vi "robot_control.vi"() -> ()   [LabVIEW 2011]
uses:
  <vilib>/Rock Robotics/WPI/DriverStation/WPI_DriverStationRobotMode.ctl
  <vilib>/Rock Robotics/WPI/Solenoid/Deprecated/WPI_SolenoidSetBool.vi
  Robot Global Data.vi
  <vilib>/Rock Robotics/WPI/Solenoid/Deprecated/WPI_SolenoidGetBool.vi
  <vilib>/addons/control/pid/pid.llb/PID (DBL).vi
  <vilib>/Rock Robotics/WPI/RobotDrive/WPI_RobotDriveArcadeDrive_Standard(NoSaturation).vi
  <vilib>/addons/control/pid/NI_PID_pid.lvlib
  <vilib>/Rock Robotics/WPI/DriverStation/DriverStationLCD/WPI_DriverStationLCDLCDLine.ctl
panel:
  out "l rate":dbl
  out "l Distance":dbl
  out "r rate":dbl
  out "r Distance":dbl
  out "w index":bool
  out "s index":bool
  in  "reinitialize":bool
  out "i per ms":dbl
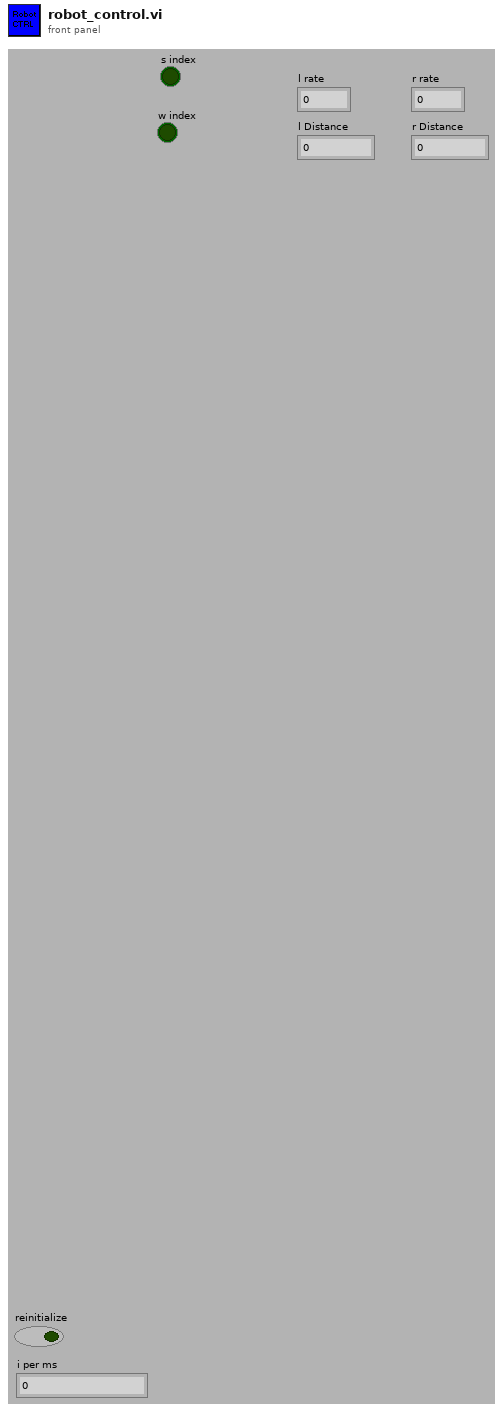
[diagram p1: front panel]
types:
  T1 = typedef "WPI_SolenoidDevRef.ctl" = cluster{"DevStatus":errorcluster, "Solenoid Module":T2, "Forward Solenoid Channel":T3, "Reverse Solenoid Channel":T3}
  T2 = typedef "FPGA_TypedefSolenoidModule.ctl" = enum16{"Solenoid Module 1", "Solenoid Module 2"}
  T3 = typedef "WPI_SolenoidChannel.ctl" = enum8{"Solenoid 1", "Solenoid 2", "Solenoid 3", "Solenoid 4", "Solenoid 5", "Solenoid 6", "Solenoid 7", "Solenoid 8", "Invalid"}
  T4 = typedef "WPI_DigitalInputDevRef.ctl" = cluster{"DevStatus":errorcluster, "DIO Channel":T5, "Digital Module":T6}
  T5 = typedef "FPGA_DIOChannel.ctl" = enum8{"DIO 1", "DIO 2", "DIO 3", "DIO 4", "DIO 5", "DIO 6", "DIO 7", "DIO 8", "DIO 9", "DIO 10", "DIO 11", "DIO 12", "DIO 13", "DIO 14", "Invalid"}
  T6 = typedef "FPGA_TypedefDigitalModule.ctl" = enum16{"Digital Module 1", "Digital Module 2"}
  T7 = typedef "WPI_EncoderDevRef.ctl" = cluster{"DevStatus":errorcluster, "EncoderIndex":T8, "CounterIndex":T9, "DistancePerCount":dbl, "Decoding Type":T10}
  T8 = typedef "FPGA_EncoderIdx.ctl" = enum8{"Enc 0", "Enc 1", "Enc 2", "Enc 3", "Invalid"}
  T9 = typedef "FPGA_CounterCtrSystemIndex.ctl" = enum8{"Ctr 0", "Ctr 1", "Ctr 2", "Ctr 3", "Ctr 4", "Ctr 5", "Ctr 6", "Ctr 7", "Invalid"}
  T10 = typedef "WPI_EncoderType.ctl" = enum16{"1x", "2x", "4x"}
  T11 = typedef "WPI_MotorControlDeviceRef.ctl" = cluster{"DeviceStatus":errorcluster, "Type":enum16{"PWM", "CAN"}, "PWM":cluster{"Digital Module":T6, "PWM Channel":T12, "DeadBand":T13}, "CAN":cluster{"Device Number":u8, "Control Mode":T14, "Semaphore":T15, "Max Vout":dbl}, "Invert":bool, "TransformRef":T16, "InvTransformRef":T16}
  T12 = typedef "FPGA_DIOPWMChannel.ctl" = enum8{"PWM 1", "PWM 2", "PWM 3", "PWM 4", "PWM 5", "PWM 6", "PWM 7", "PWM 8", "PWM 9", "PWM 10", "Invalid"}
  T13 = typedef "WPI_PWMDeadband.ctl" = cluster{"Name":string, "maxPositivePwm":i32, "minPositivePwm":i32, "centerPwm":i32, "maxNegativePwm":i32, "minNegativePwm":i32, "angularRange":u16}
  T14 = typedef "WPI_CANJaguar_ControlMode.ctl" = enum8{"Percent VBus", "Current", "Speed", "Position", "Voltage"}
  T15 = typedef "Semaphore RefNum" = refnum<k1>
  T16 = typedef "WPI_PWMTransform_ConPane.ctl" = refnum<vi>
  T17 = typedef "WPI_RobotDriveDevRef.ctl" = cluster{"DevStatus":errorcluster, "Motors[]":T11[], "Square Inputs":bool, "Max Output":dbl, "Isochronous":bool}
  T18 = typedef "WPI_DriverStationRobotMode.ctl" = enum16{"Autonomous Disabled", "Autonomous Enabled", "Teleop Disabled", "Teleop Enabled", "Timeout", "Finish"}
  T19 = typedef "WPI_DriverStationLCDLCDLine.ctl" = enum16{"Main - Line 1", "User - Line 2", "User - Line 3", "User - Line 4", "User - Line 5", "User - Line 6"}
  T20 = cluster{"proportional gain (Kc)":dbl, "integral time (Ti, min)":dbl, "derivative time (Td, min)":dbl}
  T21 = typedef "robot_control.ctl" = cluster{"Joystick1":cluster{"Buttons":T22, "Axes":cluster{"axis 1 (x)":dbl, "axis 2 (y)":dbl, "axis 3 (throttle)":dbl}}, "Joystick2":cluster{"Buttons":T22, "Axes":cluster{"axis 1 (x)":dbl, "axis 2 (y)":dbl, "axis 3 (throttle)":dbl}}, "Joystick3":cluster{"Buttons":T22, "Axes":cluster{"axis 1 (x)":dbl, "axis 2 (y)":dbl, "axis 3 (throttle)":dbl}}, "switchbox":cluster{"Driver Station Digital Input (1-8)[0]":bool, "Driver Station Digital Input (1-8)[1]":bool, "Driver Station Digital Input (1-8)[2]":bool, "Driver Station Digital Input (1-8)[3]":bool, "Driver Station Digital Input (1-8)[4]":bool, "Driver Station Digital Input (1-8)[5]":bool, "Driver Station Digital Input (1-8)[6]":bool, "Driver Station Digital Input (1-8)[7]":bool, "Driver Station Digital Input (1-8)[8]":bool}}
  T22 = typedef "WPI_JoystickButtonState.ctl" = cluster{"Button 1":bool, "Button 2":bool, "Button 3":bool, "Button 4":bool, "Button 5":bool, "Button 6":bool, "Button 7":bool, "Button 8":bool, "Button 9":bool, "Button 10":bool, "Button 11":bool, "Button 12":bool}
  T23 = typedef "match_data.ctl" = cluster{"Match Info":T24, "Derived Robot State":T25, "RobotMode":T18}
  T24 = typedef "WPI_DriverStationMatch Info.ctl" = cluster{"Autonomous Elapsed Seconds":dbl, "TeleOp Elapsed Seconds":dbl, "Disabled Elapsed Seconds":dbl, "Visited Autonomous":bool, "Visited TeleOp":bool, "Visited Disabled":bool, "Autonomous Settings":cluster{"Autonomous Style":enum16{"Iterative", "Independent"}, "VI Refnum":refnum<vi>}}
  T25 = typedef "WPI_DriverStationDerivedRobotMode.ctl" = enum16{"Init", "Execute", "Stop"}
  T26 = cluster{"Buttons":T22, "Axes":cluster{"axis 1 (x)":dbl, "axis 2 (y)":dbl, "axis 3 (throttle)":dbl}}
  T27 = cluster{"Driver Station Digital Input (1-8)[0]":bool, "Driver Station Digital Input (1-8)[1]":bool, "Driver Station Digital Input (1-8)[2]":bool, "Driver Station Digital Input (1-8)[3]":bool, "Driver Station Digital Input (1-8)[4]":bool, "Driver Station Digital Input (1-8)[5]":bool, "Driver Station Digital Input (1-8)[6]":bool, "Driver Station Digital Input (1-8)[7]":bool, "Driver Station Digital Input (1-8)[8]":bool}
  T28 = cluster{"axis 1 (x)":dbl, "axis 2 (y)":dbl, "axis 3 (throttle)":dbl}
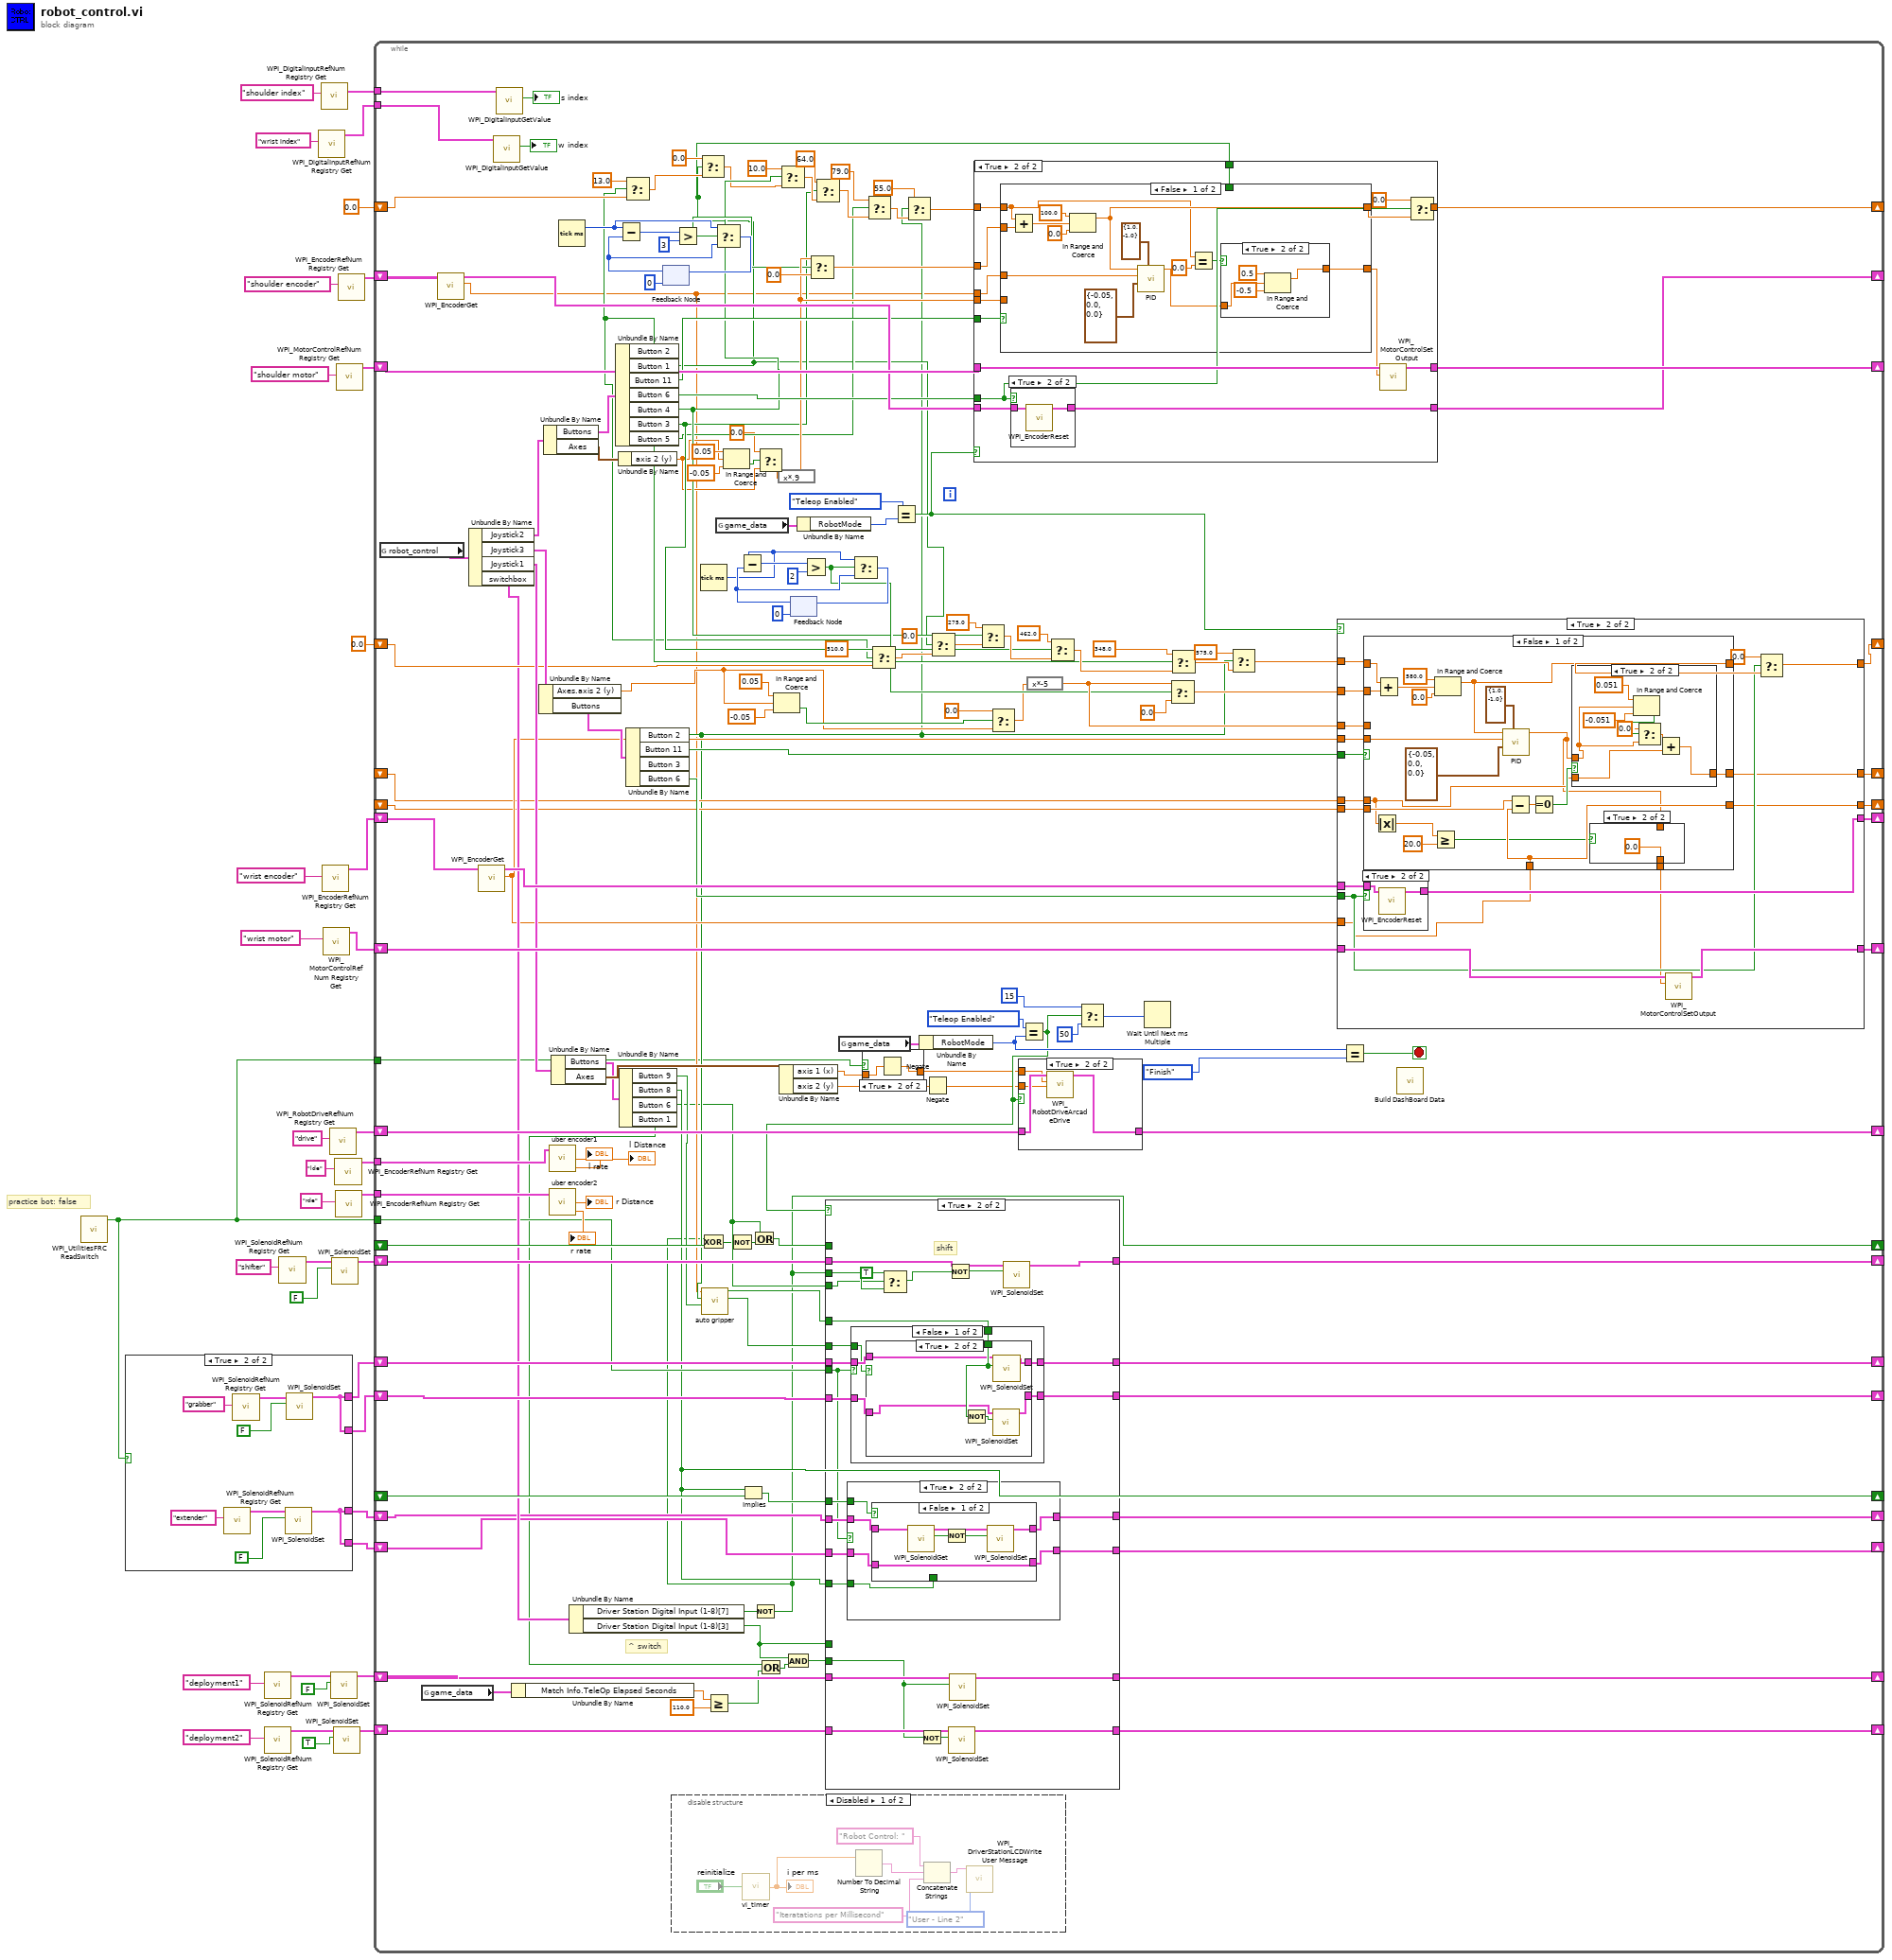
[diagram p0: block diagram]
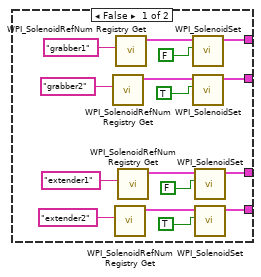
[diagram p2: hidden frame]
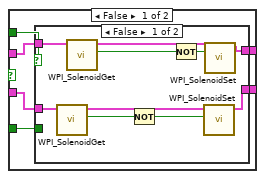
[diagram p5: hidden frame]
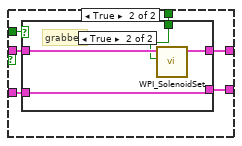
[diagram p9: hidden frame]
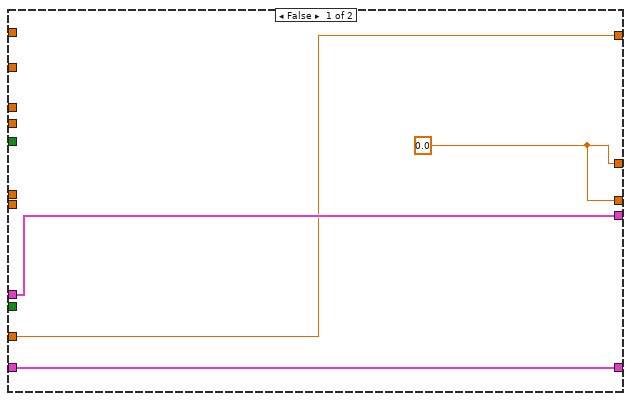
[diagram p12: hidden frame]
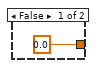
[diagram p14: hidden frame]
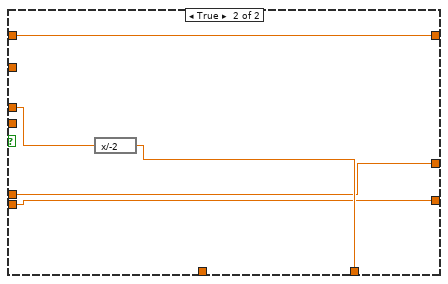
[diagram p15: hidden frame]
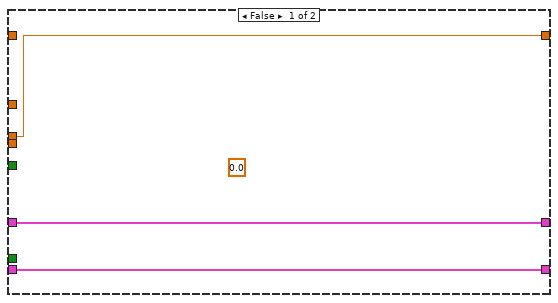
[diagram p17: hidden frame]
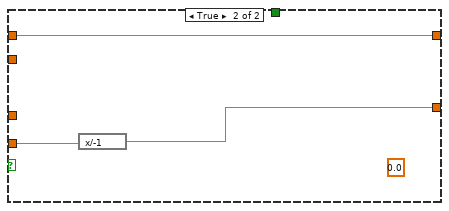
[diagram p19: hidden frame]
diagram:
  # "practice bot: false"
  n1 = call <vilib>:"WPI_UtilitiesFRC ReadSwitch.vi"() -> ("switch state"=w1:bool)  [unwired: 1 in, 10 out]
  n2 = case shown="True" w1 {
    tunnel: [w47 w55] -> w13
    tunnel: [w40 w54] -> w12
    tunnel: [w39 w55] -> w7
    tunnel: [w38 w54] -> w6
    frame False {
      n3 = call <vilib>:"WPI_SolenoidRefNum Registry Get.vi"("refnum name"="grabber2") -> ("SolenoidDevRef"=w50:T1)  [unwired: 1 in, 9 out]
      n4 = call <vilib>:"WPI_SolenoidRefNum Registry Get.vi"("refnum name"="extender2") -> ("SolenoidDevRef"=w43:T1)  [unwired: 1 in, 9 out]
      n5 = call <vilib>:"WPI_SolenoidRefNum Registry Get.vi"("refnum name"="grabber1") -> ("SolenoidDevRef"=w52:T1)  [unwired: 1 in, 9 out]
      n6 = call <vilib>:"WPI_SolenoidRefNum Registry Get.vi"("refnum name"="extender1") -> ("SolenoidDevRef"=w45:T1)  [unwired: 1 in, 9 out]
      n7 = call-poly <vilib>:"WPI_SolenoidSet.vi"("Value"=FALSE, "SolenoidDevRef"=w52) -> ("SolenoidDevRef"=w47:T1)  [unwired: 1 in, 8 out]
      n8 = call-poly <vilib>:"WPI_SolenoidSet.vi"("Value"=TRUE, "SolenoidDevRef"=w50) -> ("SolenoidDevRef"=w39:T1)  [unwired: 1 in, 8 out]
      n9 = call-poly <vilib>:"WPI_SolenoidSet.vi"("Value"=FALSE, "SolenoidDevRef"=w45) -> ("SolenoidDevRef"=w40:T1)  [unwired: 1 in, 8 out]
      n10 = call-poly <vilib>:"WPI_SolenoidSet.vi"("Value"=TRUE, "SolenoidDevRef"=w43) -> ("SolenoidDevRef"=w38:T1)  [unwired: 1 in, 8 out]
    }
    frame True {
      n11 = call <vilib>:"WPI_SolenoidRefNum Registry Get.vi"("refnum name"="extender") -> ("SolenoidDevRef"=w57:T1)  [unwired: 1 in, 9 out]
      n12 = call <vilib>:"WPI_SolenoidRefNum Registry Get.vi"("refnum name"="grabber") -> ("SolenoidDevRef"=w59:T1)  [unwired: 1 in, 9 out]
      n13 = call-poly <vilib>:"WPI_SolenoidSet.vi"("Value"=FALSE, "SolenoidDevRef"=w57) -> ("SolenoidDevRef"=w54:T1)  [unwired: 1 in, 8 out]
      n14 = call-poly <vilib>:"WPI_SolenoidSet.vi"("Value"=FALSE, "SolenoidDevRef"=w59) -> ("SolenoidDevRef"=w55:T1)  [unwired: 1 in, 8 out]
    }
  }
  n15 = call <vilib>:"WPI_SolenoidRefNum Registry Get.vi"("refnum name"="deployment1") -> ("SolenoidDevRef"=w19:T1)  [unwired: 1 in, 9 out]
  n16 = call <vilib>:"WPI_SolenoidRefNum Registry Get.vi"("refnum name"="deployment2") -> ("SolenoidDevRef"=w22:T1)  [unwired: 1 in, 9 out]
  n17 = call <vilib>:"WPI_SolenoidRefNum Registry Get.vi"("refnum name"="shifter") -> ("SolenoidDevRef"=w15:T1)  [unwired: 1 in, 9 out]
  n18 = call <vilib>:"WPI_DigitalInputRefNum Registry Get.vi"("refnum name"="wrist index") -> ("DigitalInputDevRef"=w9:T4)  [unwired: 1 in, 9 out]
  n19 = call <vilib>:"WPI_DigitalInputRefNum Registry Get.vi"("refnum name"="shoulder index") -> ("DigitalInputDevRef"=w10:T4)  [unwired: 1 in, 9 out]
  n20 = call <vilib>:"WPI_EncoderRefNum Registry Get.vi"("refnum name"="wrist encoder") -> ("EncoderDevRef"=w32:T7)  [unwired: 1 in, 9 out]
  n21 = call <vilib>:"WPI_MotorControlRefNum Registry Get.vi"("refnum name"="wrist motor") -> ("MotorControlDevRef"=w30:T11)  [unwired: 1 in, 9 out]
  n22 = call <vilib>:"WPI_RobotDriveRefNum Registry Get.vi"("refnum name"="drive") -> ("RobotDriveDevRef"=w26:T17)  [unwired: 1 in, 9 out]
  n23 = call-poly <vilib>:"WPI_SolenoidSet.vi"("Value"=FALSE, "SolenoidDevRef"=w19) -> ("SolenoidDevRef"=w18:T1)  [unwired: 1 in, 8 out]
  n24 = call-poly <vilib>:"WPI_SolenoidSet.vi"("Value"=FALSE, "SolenoidDevRef"=w15) -> ("SolenoidDevRef"=w16:T1)  [unwired: 1 in, 8 out]
  n25 = call-poly <vilib>:"WPI_SolenoidSet.vi"("Value"=TRUE, "SolenoidDevRef"=w22) -> ("SolenoidDevRef"=w20:T1)  [unwired: 1 in, 8 out]
  n26 = call <vilib>:"WPI_EncoderRefNum Registry Get.vi"("refnum name"="lde") -> ("EncoderDevRef"=w3:T7)  [unwired: 1 in, 9 out]
  n27 = call <vilib>:"WPI_EncoderRefNum Registry Get.vi"("refnum name"="rde") -> ("EncoderDevRef"=w2:T7)  [unwired: 1 in, 9 out]
  n28 = call <vilib>:"WPI_MotorControlRefNum Registry Get.vi"("refnum name"="shoulder motor") -> ("MotorControlDevRef"=w36:T11)  [unwired: 1 in, 9 out]
  n29 = call <vilib>:"WPI_EncoderRefNum Registry Get.vi"("refnum name"="shoulder encoder") -> ("EncoderDevRef"=w34:T7)  [unwired: 1 in, 9 out]
  n30 = while {
    shift-right: [w220] -> _
    shift-left: w36 -> [w221]
    shift-right: [w216] -> _
    shift-left: 0.0 ("axis 2 (y)") -> [w111]
    shift-right: [w210] -> _
    shift-left: w30 -> [w209]
    shift-right: [w208] -> _
    shift-left: 0.0 ("axis 2 (y)") -> [w107]
    shift-right: [w68] -> _
    shift-left: _ -> [w199]
    shift-right: [w78] -> _
    shift-left: _ -> [w198]
    shift-right: [w174] -> _
    shift-left: w16 -> [w196]
    shift-right: [w173] -> _
    shift-left: w13 -> [w195]
    shift-right: [w164] -> _
    shift-left: w12 -> [w80]
    shift-right: [w172] -> _
    shift-left: w18 -> [w194]
    shift-right: [w171] -> _
    shift-left: w20 -> [w193]
    shift-right: [w160] -> _
    shift-left: w26 -> [w161]
    shift-right: [w170] -> _
    shift-left: w32 -> [w212]
    shift-right: [w169] -> _
    shift-left: w34 -> [w219]
    tunnel: w10 -> [w168]
    tunnel: w9 -> [w167]
    tunnel: w1 -> [w82]
    shift-right: [w166] -> _
    shift-left: w7 -> [w165]
    shift-right: [w163] -> _
    shift-left: w6 -> [w81]
    tunnel: w3 -> [w155]
    tunnel: w2 -> [w154]
    shift-right: [w103] -> _
    shift-left: _ -> [w102]
    shift-right: [w101] -> _
    shift-left: _ -> [w100]
    tunnel: w1 -> [w65]
    stop <- w222 stop-if-true
    # "^ switch"
    n31 = global read "Robot Global Data.vi" "robot_control"() -> (w158:T21)
    n32 = global read "Robot Global Data.vi" "game_data"() -> (w77:T23)
    n33 = call <vilib>:"WPI_EncoderGet.vi"("EncoderDevRef"=w219) -> ("Distance"=w87:dbl, "EncoderDevRef"=w214:T7)  [unwired: 1 in, 8 out]
    n34 = Unbundle By Name(w158) -> ("Joystick2"=w218:T26, "Joystick3"=w213:T26, "Joystick1"=w204:T26, "switchbox"=w105:T27)
    n35 = call <vilib>:"WPI_EncoderGet.vi"("EncoderDevRef"=w212) -> ("Distance"=w104:dbl, "EncoderDevRef"=w211:T7)  [unwired: 1 in, 8 out]
    n36 = call <vilib>:"WPI_DigitalInputGetValue.vi"("DigitalInputDevRef"=w167) -> ("Value"=→"w index":bool)  [unwired: 1 in, 9 out]
    n37 = call <vilib>:"WPI_DigitalInputGetValue.vi"("DigitalInputDevRef"=w168) -> ("Value"=→"s index":bool)  [unwired: 1 in, 9 out]
    n38 = Unbundle By Name(w77) -> ("Match Info.TeleOp Elapsed Seconds"=w76:dbl)
    n39 = Unbundle By Name(w213) -> ("Axes.axis 2 (y)"=w117:dbl, "Buttons"=w118:T22)
    n40 = Unbundle By Name(w218) -> ("Buttons"=w217:T22, "Axes"=w215:T28)
    n41 = call "uber encoder1.vi"("EncoderDevRef"=w155) -> ("rate"=→"l rate":dbl, "Distance"=→"l Distance":dbl)  [unwired: 3 out]
    n42 = call "uber encoder2.vi"("EncoderDevRef"=w154) -> ("rate"=→"r rate":dbl, "Distance"=→"r Distance":dbl)  [unwired: 3 out]
    n43 = Unbundle By Name(w204) -> ("Buttons"=w202:T22, "Axes"=w203:T28)
    n44 = Tick Count (ms)() -> (millisecond timer value=w179:u32)
    n45 = Unbundle By Name(w105) -> ("Driver Station Digital Input (1-8)[7]"=w79:bool, "Driver Station Digital Input (1-8)[3]"=w73:bool)
    n46 = Unbundle By Name(w217) -> ("Button 2"=w106:bool, "Button 1"=w99:bool, "Button 11"=w201:bool, "Button 6"=w200:bool, "Button 4"=w132:bool, "Button 3"=w131:bool, "Button 5"=w130:bool)
    n47 = Unbundle By Name(w215) -> ("axis 2 (y)"=w124:dbl)
    n48 = Unbundle By Name(w202) -> ("Button 9"=w88:bool, "Button 8"=w78:bool, "Button 6"=w72:bool, "Button 1"=w62:bool)
    n49 = Select(t=13.0, s=w106, f=w111) -> (s? t:f=w110:dbl)
    n50 = Unbundle By Name(w118) -> ("Button 2"=w89:bool, "Button 11"=w197:bool, "Button 6"=w176:bool)  [unwired: 1 out]
    n51 = feedback #1(u32 0 ("millisecond timer value")) -> (w188:u32)
    n52 = Subtract(x=w179, y=w188) -> (x-y=w190:u32)
    n53 = disable-structure shown="Disabled" {
      frame Disabled {
        n54 = call "vi_timer.vi"("reinitialize"="reinitialize") -> ("ms/i"=w320:dbl)
        "i per ms" <- w320
        n55 = Number To Decimal String(number=w320) -> (decimal integer string=w322:string)  [unwired: 1 out]
        n56 = Concatenate Strings("Robot Control: " ("string"), w322, "Iteratations per Millisecond" ("string")) -> (w321:string)
        n57 = call <vilib>:"WPI_DriverStationLCDWrite User Message.vi"("line text"=w321, "line"=WPI_DriverStationLCDLCDLine."User - Line 2") -> ()  [unwired: 3 in, 11 out]
      }
      frame Enabled {
      }
    }
    n58 = Greater?(x=w190, y=u32 3) -> (0:w177:bool)
    n59 = Select(t=0.0, s=w99, f=w110) -> (s? t:f=w115:dbl)
    n60 = Tick Count (ms)() -> (millisecond timer value=w175:u32)
    n61 = call "auto gripper.vi"("button 9"=w88, "button 2"=w89, "encoder distance"=w87) -> ("change state"=w90:bool, "gripper state"=w91:bool)  [unwired: 7 out]
    n62 = Greater Or Equal?(x=w76, y=110.0) -> (x >= y?=w63:bool)
    n63 = Select(t=w179, s=w177, f=w188) -> (s? t:f=w192:u32)
    n64 = feedback-in #1(w192) -> ()
    n65 = global read "Robot Global Data.vi" "game_data"() -> (w145:T23)
    n66 = In Range and Coerce(upper limit=0.05, x=w124, lower limit=-0.05 ("upper limit")) -> (In Range?=w127:bool)  [unwired: 1 out]
    n67 = Implies(1:w198, 2:w78) -> (0:w162:bool)
    n68 = Not(x=w79) -> (.not. x?=w68:bool)
    n69 = Exclusive Or(1:w199, 2:w68) -> (0:w71:bool)
    n70 = Not(x=w71) -> (.not. x?=w70:bool)
    n71 = Or(x=w72, y=w70) -> (x .or. y?=w69:bool)
    n72 = Select(t=0.0 ("f"), s=w127, f=w124) -> (s? t:f=w126:dbl)
    n73 = Or(x=w62, y=w63) -> (x .or. y?=w64:bool)
    n74 = In Range and Coerce(upper limit=0.05, x=w117, lower limit=-0.05 ("upper limit")) -> (In Range?=w122:bool)  [unwired: 1 out]
    n75 = expression code="x*.9"(w126) -> (w185:dbl)
    n76 = Select(t=10.0, s=w132, f=w115) -> (s? t:f=w141:dbl)
    n77 = Unbundle By Name(w203) -> ("axis 1 (x)"=w66:dbl, "axis 2 (y)"=w84:dbl)
    n78 = And(x=w73, y=w64) -> (x .and. y?=w74:bool)
    n79 = feedback #2(u32 0 ("millisecond timer value")) -> (w184:u32)
    n80 = Subtract(x=w175, y=w184) -> (x-y=w182:u32)
    n81 = Unbundle By Name(w145) -> ("RobotMode"=w144:T18)
    n82 = Greater?(x=w182, y=u32 2) -> (0:w178:bool)
    n83 = Select(t=w185, s=w177, f=0.0) -> (s? t:f=w205:dbl)
    n84 = Select(t=64.0, s=w131, f=w141) -> (s? t:f=w142:dbl)
    n85 = global read "Robot Global Data.vi" "game_data"() -> (w159:T23)
    n86 = Select(t=w175, s=w178, f=w184) -> (s? t:f=w180:u32)
    n87 = feedback-in #2(w180) -> ()
    n88 = case shown="True" w65 {
      tunnel: [w224 w225] -> w67
      tunnel: w66 -> [w224 w226]
      frame False {
      }
      frame True {
        n89 = Negate(x=w226) -> (-x=w225:dbl)
      }
    }
    n90 = Select(t=79.0, s=w130, f=w142) -> (s? t:f=w94:dbl)
    n91 = Select(t=510.0, s=w106, f=w107) -> (s? t:f=w108:dbl)
    n92 = Equal?(x=WPI_DriverStationRobotMode."Teleop Enabled" ("RobotMode"), y=w144) -> (x = y?=w143:bool)
    n93 = Select(t=55.0, s=w89, f=w94) -> (s? t:f=w93:dbl)
    n94 = Unbundle By Name(w159) -> ("RobotMode"=w157:T18)
    n95 = Negate(x=w84) -> (-x=w83:dbl)
    n96 = Select(t=0.0, s=w99, f=w108) -> (s? t:f=w113:dbl)
    n97 = case shown="True" w143 {
      tunnel: w221 -> [w389 w404]
      tunnel: [w389 w403] -> w220
      tunnel: [w387 w395] -> w216
      tunnel: w87 -> [w387 w402]
      tunnel: w214 -> [w388 w400]
      tunnel: w205 -> [_ w399]
      tunnel: w201 -> [_ w398]
      tunnel: w200 -> [_ w393]
      tunnel: w185 -> [_ w391]
      tunnel: w93 -> [_ w397]
      tunnel: [w388 w396] -> w169
      tunnel: w99 -> [_ w390]
      frame False {
        (unwired) 0.0 ("axis 2 (y)")
      }
      frame True {
        n98 = case shown="False" w398 {
          tunnel: w397 -> [w405 w425]
          tunnel: [w407 w425] -> w394
          tunnel: w402 -> [w414 _]
          tunnel: w399 -> [w413 _]
          tunnel: [w410 w424] -> w401
          tunnel: w391 -> [_ w423]
          tunnel: w390 -> [_ _]
          frame False {
            n99 = Add(x=w405, y=w413) -> (x+y=w417:dbl)
            n100 = In Range and Coerce(upper limit=100.0, x=w417, lower limit=0.0) -> (coerced(x)=w407:dbl)  [unwired: 1 out]
            n101 = call-poly <vilib>:"PID.vi"("output range"=cluster{"output high":dbl, "output low":dbl} {"output high"=1.0, "output low"=-1.0}, "PID gains"=T20 {"proportional gain (Kc)"=-0.05, "integral time (Ti, min)"=0.0, "derivative time (Td, min)"=0.0}, "process variable"=w414, "setpoint"=w407) -> ("output"=w409:dbl)  [unwired: 3 in, 4 out]
            n102 = Equal?(x=w405, y=0.0) -> (x = y?=w408:bool)
            n103 = case shown="True" w408 {
              tunnel: w409 -> [w418 w421]
              tunnel: [w418 w422] -> w410
              frame False {
              }
              frame True {
                n104 = In Range and Coerce(upper limit=0.5, x=w421, lower limit=-0.5) -> (coerced(x)=w422:dbl)  [unwired: 1 out]
              }
            }
          }
          frame True {
            (unwired) 0.0 ("axis 2 (y)")
            n105 = expression code="x/-1"(w423) -> (w424:dbl)
          }
        }
        n106 = case shown="True" w393 {
          tunnel: w400 -> [w426 w428]
          tunnel: [w426 w427] -> w396
          frame False {
          }
          frame True {
            n107 = call <vilib>:"WPI_EncoderReset.vi"("EncoderDevRef"=w428) -> ("EncoderDevRef"=w427:T7)  [unwired: 1 in, 9 out]
          }
        }
        n108 = call <vilib>:"WPI_MotorControlSetOutput.vi"("Output"=w401, "MotorControlDevRef"=w404) -> ("MotorControlDevRef"=w403:T11)  [unwired: 3 in, 6 out]
        n109 = Select(t=0.0, s=w393, f=w394) -> (s? t:f=w395:dbl)
      }
    }
    n110 = Select(t=275.0, s=w132, f=w113) -> (s? t:f=w134:dbl)
    n111 = Select(t=0.0 ("f"), s=w122, f=w117) -> (s? t:f=w119:dbl)
    n112 = Equal?(x=WPI_DriverStationRobotMode."Teleop Enabled" ("RobotMode"), y=w157) -> (x = y?=w98:bool)
    n113 = case shown="True" w98 {
      tunnel: w69 -> [_ _]
      tunnel: w196 -> [w233 w259]
      tunnel: w195 -> [w231 w258]
      tunnel: w194 -> [w228 w257]
      tunnel: w193 -> [w227 w256]
      tunnel: [w233 w255] -> w174
      tunnel: [w231 w254] -> w173
      tunnel: [w228 w253] -> w172
      tunnel: [w227 w252] -> w171
      tunnel: [w232 w251] -> w166
      tunnel: w165 -> [w232 w250]
      tunnel: w80 -> [w230 w249]
      tunnel: [w230 w248] -> w164
      tunnel: w81 -> [w229 w247]
      tunnel: [w229 w246] -> w163
      tunnel: w162 -> [_ w245]
      tunnel: w82 -> [_ w244]
      tunnel: w91 -> [_ w243]
      tunnel: w90 -> [_ w242]
      tunnel: w68 -> [_ w239]
      tunnel: w78 -> [_ w241]
      tunnel: w73 -> [_ _]
      tunnel: w74 -> [_ w240]
      tunnel: w72 -> [_ w238]
      frame False {
      }
      frame True {
        # "shift"
        n114 = case shown="True" w244 {
          tunnel: w245 -> [w265 w283]
          tunnel: [w264 w282] -> w248
          tunnel: [w263 w280] -> w246
          tunnel: w247 -> [w262 w281]
          tunnel: w249 -> [w261 w279]
          tunnel: w241 -> [w260 w278]
          frame False {
            n115 = case shown="False" w265 {
              tunnel: [w275 w277] -> w264
              tunnel: [w274 w276] -> w263
              tunnel: w262 -> [w272 w276]
              tunnel: w261 -> [w273 w277]
              tunnel: w260 -> [_ _]
              frame False {
                n116 = call-poly <vilib>:"WPI_SolenoidGet.vi"("SolenoidDevRef"=w272) -> ("Value"=w267:bool, "SolenoidDevRef"=w268:T1)  [unwired: 1 in, 8 out]
                n117 = call-poly <vilib>:"WPI_SolenoidGet.vi"("SolenoidDevRef"=w273) -> ("Value"=w270:bool, "SolenoidDevRef"=w271:T1)  [unwired: 1 in, 8 out]
                n118 = Not(x=w267) -> (.not. x?=w266:bool)
                n119 = Not(x=w270) -> (.not. x?=w269:bool)
                n120 = call-poly <vilib>:"WPI_SolenoidSet.vi"("Value"=w266, "SolenoidDevRef"=w268) -> ("SolenoidDevRef"=w274:T1)  [unwired: 1 in, 8 out]
                n121 = call-poly <vilib>:"WPI_SolenoidSet.vi"("Value"=w269, "SolenoidDevRef"=w271) -> ("SolenoidDevRef"=w275:T1)  [unwired: 1 in, 8 out]
              }
              frame True {
              }
            }
          }
          frame True {
            n122 = case shown="False" w283 {
              tunnel: [w289 w290] -> w282
              tunnel: w281 -> [w287 w291]
              tunnel: [w287 w291] -> w280
              tunnel: w279 -> [w288 w290]
              tunnel: w278 -> [_ _]
              frame False {
                n123 = call-poly <vilib>:"WPI_SolenoidGet.vi"("SolenoidDevRef"=w288) -> ("Value"=w285:bool, "SolenoidDevRef"=w286:T1)  [unwired: 1 in, 8 out]
                n124 = Not(x=w285) -> (.not. x?=w284:bool)
                n125 = call-poly <vilib>:"WPI_SolenoidSet.vi"("Value"=w284, "SolenoidDevRef"=w286) -> ("SolenoidDevRef"=w289:T1)  [unwired: 1 in, 8 out]
              }
              frame True {
              }
            }
          }
        }
        n126 = case shown="False" w244 {
          tunnel: w258 -> [w294 w311]
          tunnel: [w297 w310] -> w254
          tunnel: [w296 w308] -> w251
          tunnel: w250 -> [w295 w309]
          tunnel: w243 -> [w293 w307]
          tunnel: w242 -> [w292 w306]
          frame False {
            n127 = case shown="True" w292 {
              tunnel: [w299 w304] -> w297
              tunnel: [w298 w303] -> w296
              tunnel: w295 -> [w298 w300]
              tunnel: w294 -> [w299 w301]
              tunnel: w293 -> [_ w302]
              frame False {
              }
              frame True {
                n128 = Not(x=w302) -> (.not. x?=w305:bool)
                n129 = call-poly <vilib>:"WPI_SolenoidSet.vi"("Value"=w305, "SolenoidDevRef"=w300) -> ("SolenoidDevRef"=w303:T1)  [unwired: 1 in, 8 out]
                n130 = call-poly <vilib>:"WPI_SolenoidSet.vi"("Value"=w302, "SolenoidDevRef"=w301) -> ("SolenoidDevRef"=w304:T1)  [unwired: 1 in, 8 out]
              }
            }
          }
          frame True {
            n131 = case shown="True" w306 {
              tunnel: w311 -> [w313 w315]
              tunnel: [w313 w317] -> w310
              tunnel: w309 -> [w312 w316]
              tunnel: [w312 w316] -> w308
              tunnel: w307 -> [_ w314]
              frame False {
              }
              frame True {
                # "grabber"
                n132 = call-poly <vilib>:"WPI_SolenoidSet.vi"("Value"=w314, "SolenoidDevRef"=w315) -> ("SolenoidDevRef"=w317:T1)  [unwired: 1 in, 8 out]
              }
            }
          }
        }
        n133 = Select(t=TRUE, s=w238, f=w239) -> (s? t:f=w237:bool)
        n134 = Not(x=w240) -> (.not. x?=w234:bool)
        n135 = Not(x=w237) -> (.not. x?=w236:bool)
        n136 = call-poly <vilib>:"WPI_SolenoidSet.vi"("Value"=w234, "SolenoidDevRef"=w256) -> ("SolenoidDevRef"=w252:T1)  [unwired: 1 in, 8 out]
        n137 = call-poly <vilib>:"WPI_SolenoidSet.vi"("Value"=w240, "SolenoidDevRef"=w257) -> ("SolenoidDevRef"=w253:T1)  [unwired: 1 in, 8 out]
        n138 = call-poly <vilib>:"WPI_SolenoidSet.vi"("Value"=w236, "SolenoidDevRef"=w259) -> ("SolenoidDevRef"=w255:T1)  [unwired: 1 in, 8 out]
      }
    }
    n139 = case shown="True" w98 {
      tunnel: w161 -> [w429 w433]
      tunnel: [w429 w432] -> w160
      tunnel: w83 -> [_ w431]
      tunnel: w67 -> [_ w430]
      frame False {
      }
      frame True {
        n140 = call-poly <vilib>:"WPI_RobotDriveArcadeDrive.vi"("Y axis value"=w431, "X axis value"=w430, "RobotDriveDevRef"=w433) -> ("RobotDriveDevRef"=w432:T17)  [unwired: 1 in, 7 out]
      }
    }
    n141 = expression code="x*-5"(w119) -> (w186:dbl)
    n142 = Select(t=462.0, s=w131, f=w134) -> (s? t:f=w133:dbl)
    n143 = Select(t=u32 15 ("millisecond timer value"), s=w98, f=u32 50 ("millisecond timer value")) -> (s? t:f=w149:u32)
    n144 = Wait Until Next ms Multiple(millisecond multiple=w149) -> ()  [unwired: 1 out]
    n145 = Select(t=w186, s=w178, f=0.0) -> (s? t:f=w187:dbl)
    n146 = Select(t=348.0, s=w130, f=w133) -> (s? t:f=w97:dbl)
    n147 = Select(t=575.0, s=w89, f=w97) -> (s? t:f=w96:dbl)
    n148 = case shown="True" w143 {
      tunnel: w211 -> [w328 w347]
      tunnel: w104 -> [_ w346]
      tunnel: [w327 w345] -> w210
      tunnel: w209 -> [w327 w344]
      tunnel: [w325 w337] -> w208
      tunnel: w197 -> [_ w343]
      tunnel: w187 -> [_ w342]
      tunnel: w186 -> [_ w341]
      tunnel: w96 -> [_ w340]
      tunnel: w176 -> [_ w335]
      tunnel: [w328 w339] -> w170
      tunnel: w104 -> [w325 w333]
      tunnel: [w326 w332] -> w103
      tunnel: w102 -> [_ w331]
      tunnel: [w326 w330] -> w101
      tunnel: w100 -> [_ w329]
      frame False {
        w326 = 0.0 ("axis 2 (y)")
      }
      frame True {
        n149 = case shown="False" w343 {
          tunnel: w340 -> [w367 w383]
          tunnel: [w360 w383] -> w336
          tunnel: w346 -> [w363 _]
          tunnel: w341 -> [_ w382]
          tunnel: w342 -> [w359 _]
          tunnel: [w350 w381] -> w334
          tunnel: w333 -> [w358 _]
          tunnel: [w354 w380] -> w332
          tunnel: w331 -> [w351 w380]
          tunnel: [w358 w379] -> w330
          tunnel: w329 -> [w357 w379]
          frame False {
            n150 = Absolute Value(x=w351) -> (abs(x)=w348:dbl)
            n151 = Add(x=w367, y=w359) -> (x+y=w366:dbl)
            n152 = Greater Or Equal?(x=w348, y=20.0) -> (x >= y?=w353:bool)
            n153 = In Range and Coerce(upper limit=580.0, x=w366, lower limit=0.0) -> (coerced(x)=w360:dbl)  [unwired: 1 out]
            n154 = call-poly <vilib>:"PID.vi"("output range"=cluster{"output high":dbl, "output low":dbl} {"output high"=1.0, "output low"=-1.0}, "PID gains"=T20 {"proportional gain (Kc)"=-0.05, "integral time (Ti, min)"=0.0, "derivative time (Td, min)"=0.0}, "process variable"=w363, "setpoint"=w360) -> ("output"=w349:dbl)  [unwired: 3 in, 4 out]
            n155 = Subtract(x=w357, y=w358) -> (x-y=w356:dbl)
            n156 = Equal To 0?(x=w356) -> (x = 0?=w355:bool)
            n157 = case shown="True" w355 {
              tunnel: w349 -> [_ w371]
              tunnel: [0.0 w377] -> w354
              tunnel: w351 -> [_ w378]
              frame False {
              }
              frame True {
                n158 = In Range and Coerce(upper limit=0.051, x=w371, lower limit=-0.051 ("upper limit")) -> (In Range?=w374:bool)  [unwired: 1 out]
                n159 = Select(t=0.0, s=w374, f=w371) -> (s? t:f=w373:dbl)
                n160 = Add(x=w373, y=w378) -> (x+y=w377:dbl)
              }
            }
            n161 = case shown="True" w353 {
              tunnel: [w368 0.0] -> w350
              tunnel: w349 -> [w368 _]
              frame False {
              }
              frame True {
              }
            }
          }
          frame True {
            n162 = expression code="x/-2"(w382) -> (w381:dbl)
          }
        }
        n163 = case shown="True" w335 {
          tunnel: w347 -> [w384 w386]
          tunnel: [w384 w385] -> w339
          frame False {
          }
          frame True {
            n164 = call <vilib>:"WPI_EncoderReset.vi"("EncoderDevRef"=w386) -> ("EncoderDevRef"=w385:T7)  [unwired: 1 in, 9 out]
          }
        }
        n165 = call <vilib>:"WPI_MotorControlSetOutput.vi"("Output"=w334, "MotorControlDevRef"=w344) -> ("MotorControlDevRef"=w345:T11)  [unwired: 3 in, 6 out]
        n166 = Select(t=0.0, s=w335, f=w336) -> (s? t:f=w337:dbl)
      }
    }
    n167 = Equal?(x=w157, y=WPI_DriverStationRobotMode."Finish" ("RobotMode")) -> (x = y?=w222:bool)
    n168 = call "Build DashBoard Data.vi"() -> ()  [unwired: 1 in, 11 out]
  }
